vi "Get Result of the Proccess from URL link.vi"(8 "error in":errorcluster, 9 "Proccess":string, 10 "Serial number":string, 11 "Model":string) -> (0 "error out":errorcluster, 3 "Result of the Proccess":string)   [LabVIEW 2025, in "MES Interlcok.lvlib"]
uses:
  MES Interlcok.lvlib
  <vilib>/httpClient/LabVIEWHTTPClient.lvlib
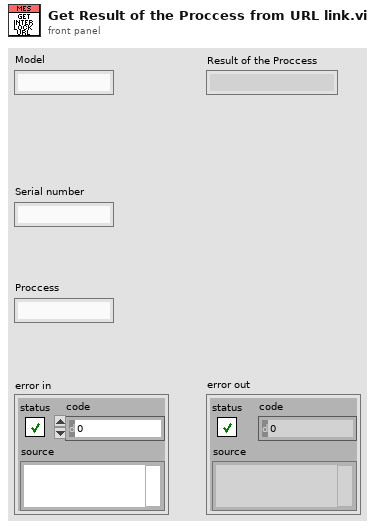
[diagram p1: front panel]
types:
  T1 = typedef "LabVIEWHTTPClient.lvlib/ClientHandle.ctl" = refnum<k1>
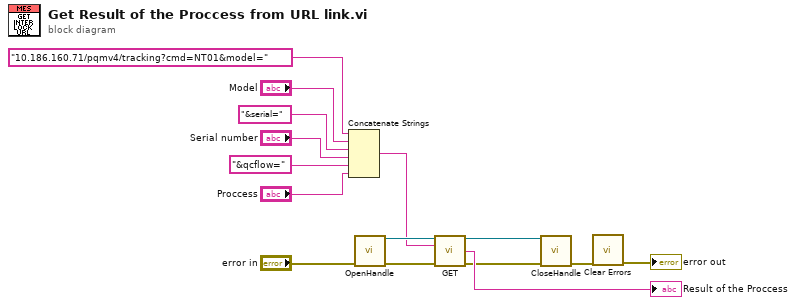
[diagram p0: block diagram]
diagram:
  n1 = Concatenate Strings("10.186.160.71/pqmv4/tracking?cmd=NT01&model=", "Model", "&serial=", "Serial number", "&qcflow=", "Proccess") -> (w3:string)
  n2 = call <vilib>:"OpenHandle.vi"("error in (no error)"="error in") -> ("client handle out"=w15:T1, "error out"=w14:errorcluster)  [unwired: 13 in]
  n3 = call <vilib>:"GET.vi"("client handle"=w15, "url"=w3, "error in (no error)"=w14) -> ("client handle out"=w12:T1, "body"=→"Result of the Proccess":string, "error out"=w11:errorcluster)  [unwired: 9 in, 1 out]
  n4 = call <vilib>:"CloseHandle.vi"("client handle"=w12, "error in (no error)"=w11) -> ("error out"=w2:errorcluster)  [unwired: 13 in]
  n5 = call <vilib>:"Clear Errors.vi"("error in (no error)"=w2) -> ("error out"=→"error out":errorcluster)  [unwired: 5 in, 1 out]
